vi "Configure 1154A Probe.vi"(7 "Amplifier Gain (0: X1)":i32(ring) items=["X1", "X10"], 8 "error in (no error)":errorcluster, 9 "Amplifier Attenuation (0: Divide by 1)":i32(ring) items=["Divide by 1", "Divide by 10"], 10 "Channel (1: Channel 1)":i32(ring)=1 items=["Channel 1"=1, "Channel 2"=2, "Channel 3"=3, "Channel 4"=4], 11 "VISA resource name":refnum<visa-resource-name>) -> (0 "error out":errorcluster, 3 "VISA resource name out":refnum<visa-resource-name>)   [LabVIEW 2013, in "Agilent 90000 Series.lvlib"]
doc: "Configures the 1154A probe's settings."
uses:
  Agilent 90000 Series.lvlib
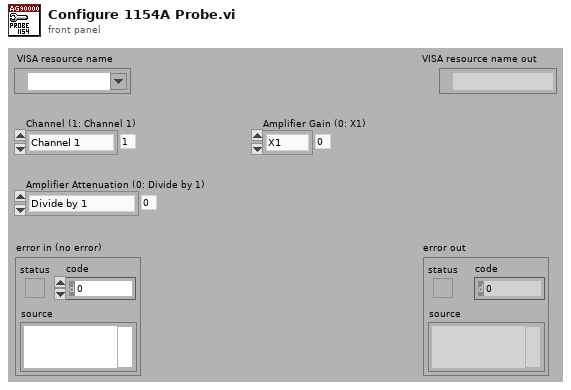
[diagram p1: front panel]
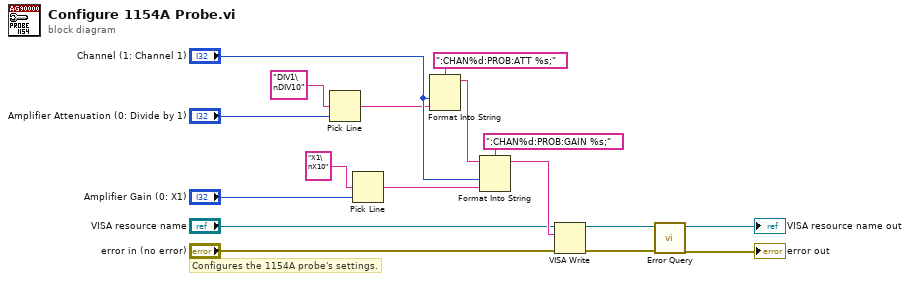
[diagram p0: block diagram]
diagram:
  # "Configures the 1154A probe's settings."
  n1 = Pick Line(multi-line string="DIV1\nDIV10", line index="Amplifier Attenuation (0: Divide by 1)") -> (output string=w13:string)  [unwired: 1 out]
  n2 = Pick Line(multi-line string="X1\nX10", line index="Amplifier Gain (0: X1)") -> (output string=w8:string)  [unwired: 1 out]
  n3 = Format Into String(format string=":CHAN%d:PROB:ATT %s;", "Channel (1: Channel 1)", w13) -> (resulting string=w10:string)  [unwired: 2 in, 1 out]
  n4 = Format Into String(format string=":CHAN%d:PROB:GAIN %s;", initial string=w10, "Channel (1: Channel 1)", w8) -> (resulting string=w7:string)  [unwired: 1 in, 1 out]
  n5 = VISA Write(VISA resource name="VISA resource name", write buffer=w7, error in (no error)="error in (no error)") -> (VISA resource name out=w4:refnum<visa-resource-name>, error out=w3:errorcluster)  [unwired: 1 out]
  n6 = call "Error Query.vi"("error in (no error)"=w3, "VISA resource name"=w4) -> ("error out"=→"error out":errorcluster, "VISA resource name out"=→"VISA resource name out":refnum<visa-resource-name>)  [unwired: 8 out]
